vi "Valve_Read.vi"(7 "In Array":fxp<+/-,64,32>[](array[numeric])) -> (0 "Valve 4":dbl, 1 "Valve 3":dbl, 2 "Valve 2":dbl, 3 "Valve 1":dbl)   [LabVIEW 2014]
panel:
  out "x/y 2":dbl
  out "x/y":dbl
  out "(hi.lo)":u16
  # "Valve Read Vi V190213"
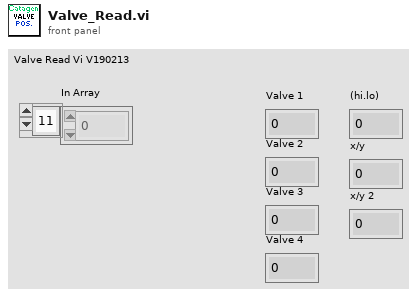
[diagram p1: front panel]
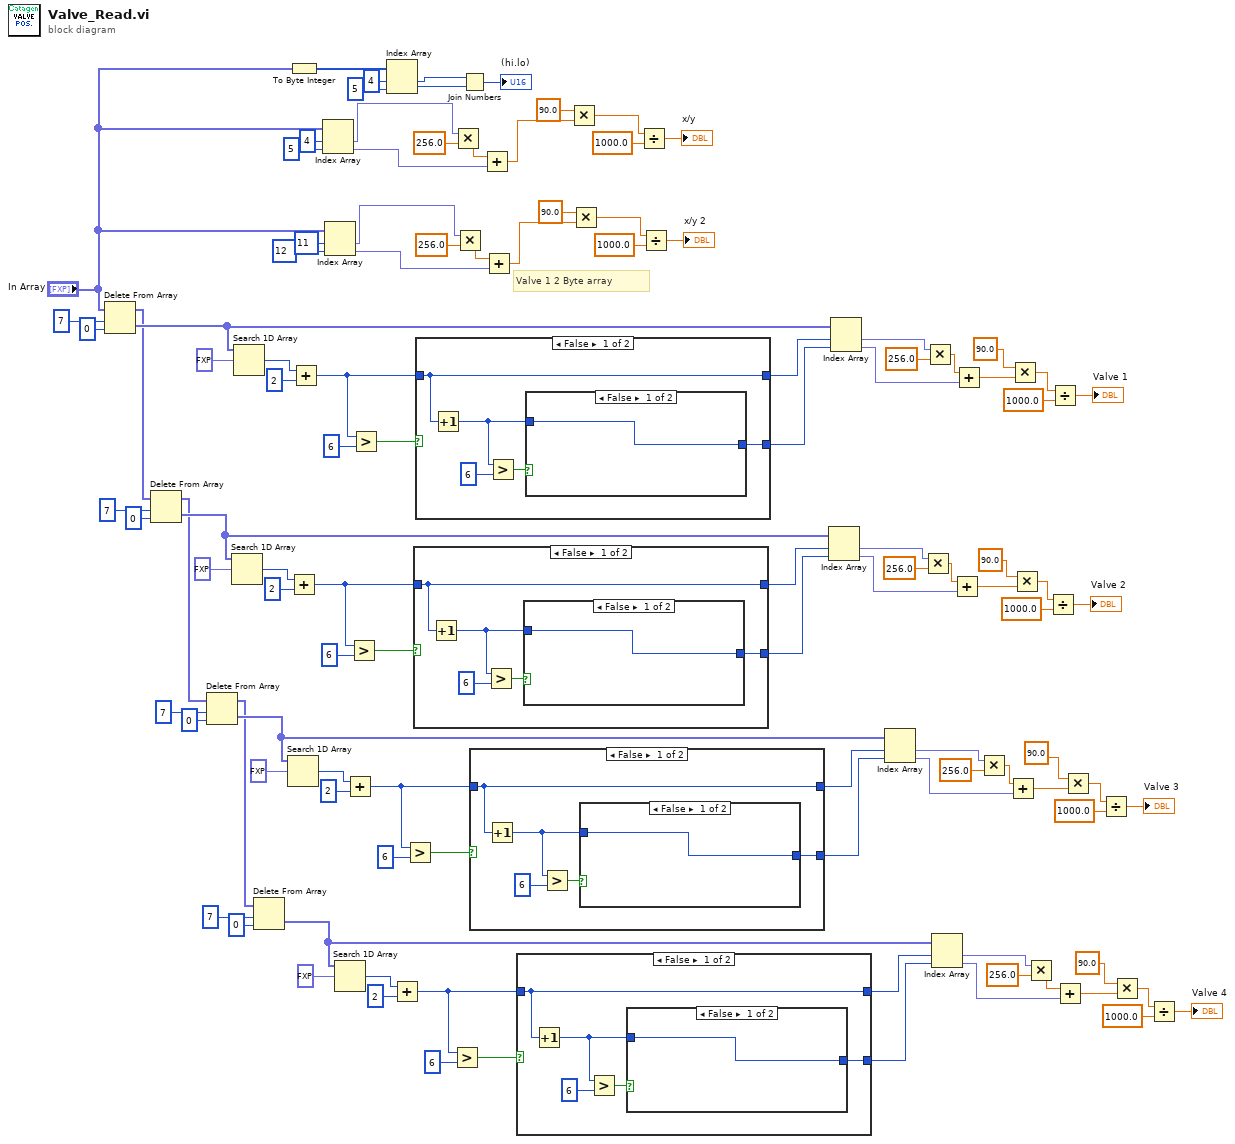
[diagram p0: block diagram]
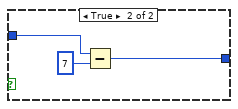
[diagram p2: hidden frame]
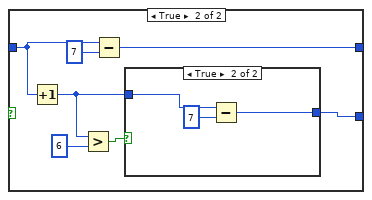
[diagram p3: hidden frame]
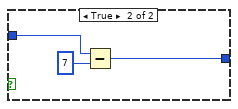
[diagram p5: hidden frame]
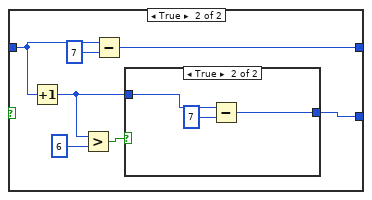
[diagram p6: hidden frame]
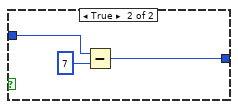
[diagram p8: hidden frame]
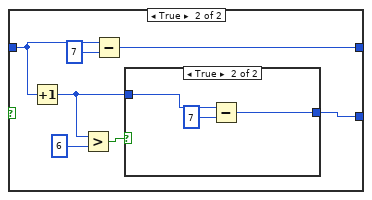
[diagram p9: hidden frame]
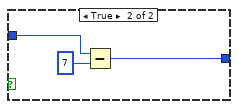
[diagram p11: hidden frame]
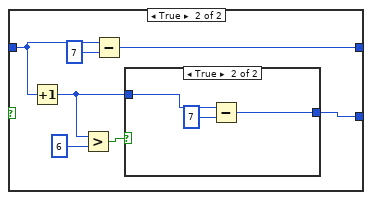
[diagram p12: hidden frame]
diagram:
  # "Valve 1 2 Byte array"
  n1 = Delete From Array(array="In Array", length=7, index=0) -> (deleted portion=w75:fxp<+/-,64,32>[], array with subset deleted=w43:fxp<+/-,64,32>[])
  n2 = Delete From Array(array=w43, length=7, index=0) -> (deleted portion=w44:fxp<+/-,64,32>[], array with subset deleted=w22:fxp<+/-,64,32>[])
  n3 = Delete From Array(array=w22, length=7, index=0) -> (deleted portion=w42:fxp<+/-,64,32>[], array with subset deleted=w1:fxp<+/-,64,32>[])
  n4 = Search 1D Array(1D array=w44, element=fxp<+/-,64,32> 4.0) -> (index of element=w48:i32)  [unwired: 1 in]
  n5 = Search 1D Array(1D array=w75, element=fxp<+/-,64,32> 4.0) -> (index of element=w80:i32)  [unwired: 1 in]
  n6 = Delete From Array(array=w1, length=7, index=0) -> (deleted portion=w2:fxp<+/-,64,32>[])  [unwired: 1 out]
  n7 = Search 1D Array(1D array=w42, element=fxp<+/-,64,32> 4.0) -> (index of element=w38:i32)  [unwired: 1 in]
  n8 = To Byte Integer(number="In Array") -> (8bit integer=w108:i8[])
  n9 = Add(x=w48, y=2) -> (x+y=w51:i32)
  n10 = Add(x=w80, y=2) -> (x+y=w77:i32)
  n11 = Index Array(array="In Array", index #1=4 ("index"), index #2=5 ("index")) -> (element #1=w103:fxp<+/-,64,32>, element #2=w102:fxp<+/-,64,32>)
  n12 = Index Array(array="In Array", index #1=11 ("index"), index #2=12 ("index")) -> (element #1=w88:fxp<+/-,64,32>, element #2=w89:fxp<+/-,64,32>)
  n13 = Search 1D Array(1D array=w2, element=fxp<+/-,64,32> 4.0) -> (index of element=w6:i32)  [unwired: 1 in]
  n14 = Add(x=w38, y=2) -> (x+y=w35:i32)
  n15 = Greater?(x=w51, y=6) -> (0:w52:bool)
  n16 = Greater?(x=w77, y=6) -> (0:w76:bool)
  n17 = Index Array(array=w108, index #1=4 ("index"), index #2=5 ("index")) -> (element #1=w107:i8, element #2=w106:i8)
  n18 = Add(x=w6, y=2) -> (x+y=w9:i32)
  n19 = Greater?(x=w35, y=6) -> (0:w34:bool)
  n20 = case shown="False" w52 {
    tunnel: w51 -> [w117 w125]
    tunnel: [w117 w126] -> w53
    tunnel: [w113 w122] -> w54
    frame False {
      n21 = Increment(x=w117) -> (x+1=w114:i32)
      n22 = Greater?(x=w114, y=6) -> (0:w116:bool)
      n23 = case shown="False" w116 {
        tunnel: w114 -> [w118 w121]
        tunnel: [w118 w119] -> w113
        frame False {
        }
        frame True {
          n24 = Subtract(x=w121, y=7) -> (x-y=w119:i32)
        }
      }
    }
    frame True {
      n25 = Increment(x=w125) -> (x+1=w123:i32)
      n26 = Greater?(x=w123, y=6) -> (0:w128:bool)
      n27 = Subtract(x=w125, y=7) -> (x-y=w126:i32)
      n28 = case shown="True" w128 {
        tunnel: w123 -> [w129 w132]
        tunnel: [w129 w131] -> w122
        frame False {
        }
        frame True {
          n29 = Subtract(x=w132, y=7) -> (x-y=w131:i32)
        }
      }
    }
  }
  n30 = case shown="False" w76 {
    tunnel: w77 -> [w137 w145]
    tunnel: [w137 w146] -> w74
    tunnel: [w133 w142] -> w73
    frame False {
      n31 = Increment(x=w137) -> (x+1=w134:i32)
      n32 = Greater?(x=w134, y=6) -> (0:w136:bool)
      n33 = case shown="False" w136 {
        tunnel: w134 -> [w138 w141]
        tunnel: [w138 w139] -> w133
        frame False {
        }
        frame True {
          n34 = Subtract(x=w141, y=7) -> (x-y=w139:i32)
        }
      }
    }
    frame True {
      n35 = Increment(x=w145) -> (x+1=w143:i32)
      n36 = Greater?(x=w143, y=6) -> (0:w148:bool)
      n37 = Subtract(x=w145, y=7) -> (x-y=w146:i32)
      n38 = case shown="True" w148 {
        tunnel: w143 -> [w149 w152]
        tunnel: [w149 w151] -> w142
        frame False {
        }
        frame True {
          n39 = Subtract(x=w152, y=7) -> (x-y=w151:i32)
        }
      }
    }
  }
  n40 = Greater?(x=w9, y=6) -> (0:w10:bool)
  n41 = Multiply(x=w103, y=256.0) -> (x*y=w101:dbl)
  n42 = Multiply(x=w88, y=256.0) -> (x*y=w90:dbl)
  n43 = Join Numbers(hi=w107, lo=w106) -> ((hi.lo)=→"(hi.lo)":u16)
  n44 = case shown="False" w34 {
    tunnel: w35 -> [w157 w165]
    tunnel: [w157 w166] -> w33
    tunnel: [w153 w162] -> w32
    frame False {
      n45 = Increment(x=w157) -> (x+1=w154:i32)
      n46 = Greater?(x=w154, y=6) -> (0:w156:bool)
      n47 = case shown="False" w156 {
        tunnel: w154 -> [w158 w161]
        tunnel: [w158 w159] -> w153
        frame False {
        }
        frame True {
          n48 = Subtract(x=w161, y=7) -> (x-y=w159:i32)
        }
      }
    }
    frame True {
      n49 = Increment(x=w165) -> (x+1=w163:i32)
      n50 = Greater?(x=w163, y=6) -> (0:w168:bool)
      n51 = Subtract(x=w165, y=7) -> (x-y=w166:i32)
      n52 = case shown="True" w168 {
        tunnel: w163 -> [w169 w172]
        tunnel: [w169 w171] -> w162
        frame False {
        }
        frame True {
          n53 = Subtract(x=w172, y=7) -> (x-y=w171:i32)
        }
      }
    }
  }
  n54 = Add(x=w101, y=w102) -> (x+y=w100:dbl)
  n55 = Add(x=w90, y=w89) -> (x+y=w91:dbl)
  n56 = case shown="False" w10 {
    tunnel: w9 -> [w177 w185]
    tunnel: [w177 w186] -> w11
    tunnel: [w173 w182] -> w12
    frame False {
      n57 = Increment(x=w177) -> (x+1=w174:i32)
      n58 = Greater?(x=w174, y=6) -> (0:w176:bool)
      n59 = case shown="False" w176 {
        tunnel: w174 -> [w178 w181]
        tunnel: [w178 w179] -> w173
        frame False {
        }
        frame True {
          n60 = Subtract(x=w181, y=7) -> (x-y=w179:i32)
        }
      }
    }
    frame True {
      n61 = Increment(x=w185) -> (x+1=w183:i32)
      n62 = Greater?(x=w183, y=6) -> (0:w188:bool)
      n63 = Subtract(x=w185, y=7) -> (x-y=w186:i32)
      n64 = case shown="True" w188 {
        tunnel: w183 -> [w189 w192]
        tunnel: [w189 w191] -> w182
        frame False {
        }
        frame True {
          n65 = Subtract(x=w192, y=7) -> (x-y=w191:i32)
        }
      }
    }
  }
  n66 = Multiply(x=90.0, y=w100) -> (x*y=w99:dbl)
  n67 = Multiply(x=90.0, y=w91) -> (x*y=w92:dbl)
  n68 = Divide(x=w99, y=1000.0) -> (x/y=→"x/y":dbl)
  n69 = Divide(x=w92, y=1000.0) -> (x/y=→"x/y 2":dbl)
  n70 = Index Array(array=w44, index #1=w53, index #2=w54) -> (element #1=w61:fxp<+/-,64,32>, element #2=w62:fxp<+/-,64,32>)
  n71 = Index Array(array=w75, index #1=w74, index #2=w73) -> (element #1=w66:fxp<+/-,64,32>, element #2=w65:fxp<+/-,64,32>)
  n72 = Index Array(array=w42, index #1=w33, index #2=w32) -> (element #1=w25:fxp<+/-,64,32>, element #2=w24:fxp<+/-,64,32>)
  n73 = Multiply(x=w61, y=256.0) -> (x*y=w59:dbl)
  n74 = Multiply(x=w66, y=256.0) -> (x*y=w68:dbl)
  n75 = Index Array(array=w2, index #1=w11, index #2=w12) -> (element #1=w19:fxp<+/-,64,32>, element #2=w20:fxp<+/-,64,32>)
  n76 = Add(x=w59, y=w62) -> (x+y=w58:dbl)
  n77 = Add(x=w68, y=w65) -> (x+y=w69:dbl)
  n78 = Multiply(x=w25, y=256.0) -> (x*y=w27:dbl)
  n79 = Add(x=w27, y=w24) -> (x+y=w28:dbl)
  n80 = Multiply(x=90.0, y=w69) -> (x*y=w70:dbl)
  n81 = Multiply(x=90.0, y=w58) -> (x*y=w57:dbl)
  n82 = Multiply(x=w19, y=256.0) -> (x*y=w17:dbl)
  n83 = Divide(x=w57, y=1000.0) -> (x/y=→"Valve 2":dbl)
  n84 = Divide(x=w70, y=1000.0) -> (x/y=→"Valve 1":dbl)
  n85 = Add(x=w17, y=w20) -> (x+y=w16:dbl)
  n86 = Multiply(x=90.0, y=w28) -> (x*y=w29:dbl)
  n87 = Divide(x=w29, y=1000.0) -> (x/y=→"Valve 3":dbl)
  n88 = Multiply(x=90.0, y=w16) -> (x*y=w15:dbl)
  n89 = Divide(x=w15, y=1000.0) -> (x/y=→"Valve 4":dbl)
